vi "ProceedProcessSelection_backup.vi"(7 "ParamInput":variant, 8 "error in (no error)":errorcluster, 9 "Process_Type":T1, 10 "queue in":refnum<queue>, 11 "TabControl in":refnum<vi>) -> (0 "Error Out":errorcluster)   [LabVIEW 2015]
uses:
  Controls/Process_UIAction.ctl
  Controls/Process_Type.ctl
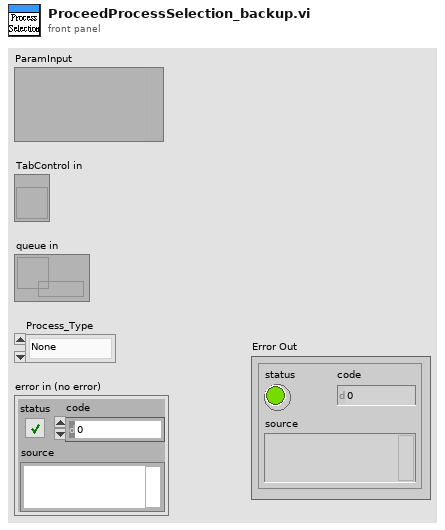
[diagram p1: front panel]
types:
  T1 = typedef "Process_Type.ctl" = enum16{"None", "ExtractPlane", "BinaryMono", "Operators", "GrayMorphology", "Filters", "Lookup Table", "Particle Filter", "Mask"}
  T2 = typedef "Process_UIAction.ctl" = cluster{"Process_UIActionCmd":enum16{"Init", "SingleStep", "RunAllSteps", "RemoveSteps", "PreTest", "Exist"}, "Process_UIParam":variant, "EventName":string}
  T3 = typedef "Process_UIAction.ctl" = cluster{"Process_UIActionCmd":enum16{"Init", "SingleStep", "RunPreviousStpes", "RunAllSteps", "RemoveSteps", "Exist"}, "Process_UIParam":variant, "EventName":string}
  T4 = typedef "UI_Process_Type.ctl" = enum32{"None", "ExtractPlane", "BinaryMono", "Operators"}
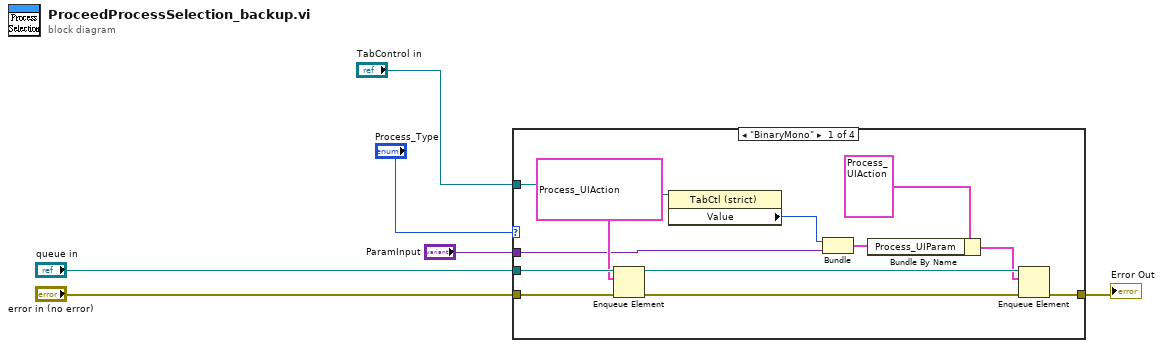
[diagram p0: block diagram]
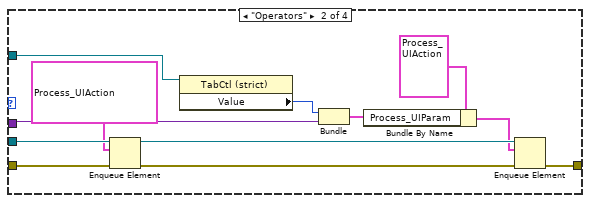
[diagram p2: hidden frame]
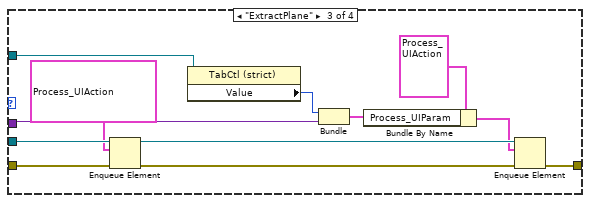
[diagram p3: hidden frame]
diagram:
  n1 = case shown="\"BinaryMono\"" "Process_Type" {
    tunnel: "queue in" -> [w18 w30 w42 _]
    tunnel: "error in (no error)" -> [w17 w29 w41 w43]
    tunnel: "TabControl in" -> [w9 w21 w33 _]
    tunnel: "ParamInput" -> [w8 w20 w32 _]
    tunnel: [w7 w19 w31 w43] -> w1
    frame "BinaryMono" {
      n2 = Enqueue Element(queue=w18, element=T3 {"Process_UIActionCmd"=enum."RunPreviousStpes", "Process_UIParam"=variant, "EventName"=""}, error in (no error)=w17) -> (queue out=w15:refnum<queue>, error out=w14:errorcluster)  [unwired: 1 in, 1 out]
      n3 = property on="Property Node" class="TabCtl (strict)"(reference=w9) -> ("Value"=w11:T4)  [unwired: 1 in, 2 out]
      n4 = Bundle("Value"=w11, "ParamInput"=w8) -> (w10:cluster{"Value":T4, "ParamInput":variant})  [unwired: 1 in]
      n5 = Bundle By Name(cluster=T2 {"Process_UIActionCmd"=enum."SingleStep", "Process_UIParam"=variant, "EventName"=""} ("element"), "Process_UIParam"=w10) -> (w12:T2)
      n6 = Enqueue Element(queue=w15, element=w12, error in (no error)=w14) -> (error out=w7:errorcluster)  [unwired: 1 in, 2 out]
    }
    frame "Operators" {
      n7 = Enqueue Element(queue=w30, element=T3 {"Process_UIActionCmd"=enum."RunPreviousStpes", "Process_UIParam"=variant, "EventName"=""}, error in (no error)=w29) -> (queue out=w27:refnum<queue>, error out=w26:errorcluster)  [unwired: 1 in, 1 out]
      n8 = property on="Property Node" class="TabCtl (strict)"(reference=w21) -> ("Value"=w23:T4)  [unwired: 1 in, 2 out]
      n9 = Bundle("Value"=w23, "ParamInput"=w20) -> (w22:cluster{"Value":T4, "ParamInput":variant})  [unwired: 1 in]
      n10 = Bundle By Name(cluster=T2 {"Process_UIActionCmd"=enum."SingleStep", "Process_UIParam"=variant, "EventName"=""} ("element"), "Process_UIParam"=w22) -> (w24:T2)
      n11 = Enqueue Element(queue=w27, element=w24, error in (no error)=w26) -> (error out=w19:errorcluster)  [unwired: 1 in, 2 out]
    }
    frame "ExtractPlane" {
      n12 = Enqueue Element(queue=w42, element=T3 {"Process_UIActionCmd"=enum."RunPreviousStpes", "Process_UIParam"=variant, "EventName"=""}, error in (no error)=w41) -> (queue out=w39:refnum<queue>, error out=w38:errorcluster)  [unwired: 1 in, 1 out]
      n13 = property on="Property Node" class="TabCtl (strict)"(reference=w33) -> ("Value"=w35:T4)  [unwired: 1 in, 2 out]
      n14 = Bundle("Value"=w35, "ParamInput"=w32) -> (w34:cluster{"Value":T4, "ParamInput":variant})  [unwired: 1 in]
      n15 = Bundle By Name(cluster=T2 {"Process_UIActionCmd"=enum."SingleStep", "Process_UIParam"=variant, "EventName"=""} ("element"), "Process_UIParam"=w34) -> (w36:T2)
      n16 = Enqueue Element(queue=w39, element=w36, error in (no error)=w38) -> (error out=w31:errorcluster)  [unwired: 1 in, 2 out]
    }
    frame "None", Default {
    }
  }
  "Error Out" <- w1
